vi "Follower Setter.vi"(0 "DeviceReference":T1, 3 "Update Frequency (Hz)":dbl=100.0, 5 "MasterID":i32, 7 "OpposeMasterDirection":bool) -> (4 "DeviceReference Out":T1)   [LabVIEW 2020]
doc: "Follow the motor output of another Talon.\nIf Talon is in torque control, the torque is copied - which will increase the total torque applied. If Talon is in percent supply output control, the duty cycle is matched. Motor direction either matches master's configured direction or opposes it based on OpposeMasterDirection."
uses:
  DeviceReference.ctl
  <userlib>/CTRE_PhoenixTools/CTRE_PhoenixTools.lvlib
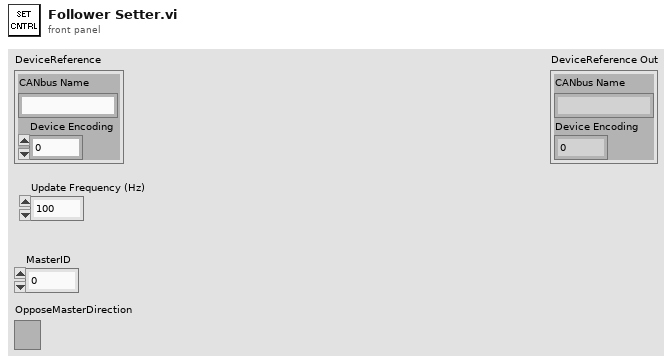
[diagram p1: front panel]
types:
  T1 = typedef "DeviceReference.ctl" = cluster{"CANbus Name":string, "Device Encoding":u32}
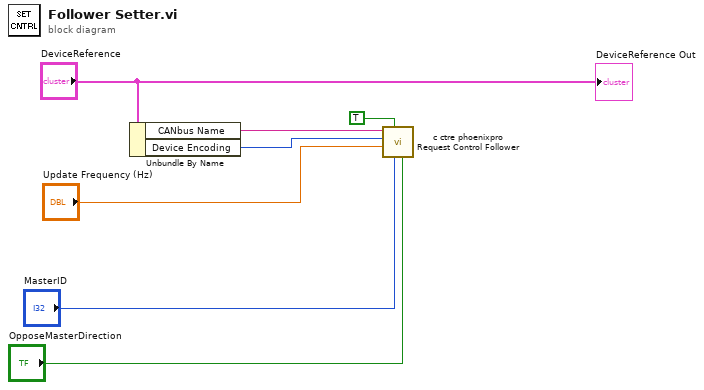
[diagram p0: block diagram]
diagram:
  n1 = Unbundle By Name("DeviceReference") -> ("CANbus Name"=w6:string, "Device Encoding"=w5:u32)
  n2 = call <userlib>:"c ctre phoenixpro Request Control Follower.vi"("OpposeMasterDirection"="OpposeMasterDirection", "MasterID"="MasterID", "cancelOtherRequests"=TRUE, "updateTime"="Update Frequency (Hz)", "ecuEncoding"=w5, "canbus"=w6) -> ()  [unwired: 4 in, 2 out]
  "DeviceReference Out" <- "DeviceReference"
